vi "USRP Dummy DMA Fixed Fetch (Host).vi"() -> ()   [LabVIEW 2016]
uses:
  <vilib>/userdefined/High Color/nirio_resource_hc.ctl
  <vilib>/FPGAPlugInAG/USRP 294xR; 295xR 200 MSps/niLvFpga_Open_USRP 294xR; 295xR 200 MSps.vi
  <vilib>/rvi/interface/common/dynamic/niFpgaDynamicAddResources.vi
  <vilib>/FPGAPlugInAG/Dynamic/niLvFpga_Download_Dynamic.vi
  <vilib>/FPGAPlugInAG/Dynamic/niLvFpga_Run_Dynamic.vi
  <vilib>/Utility/error.llb/Error Cluster From Error Code.vi
  <vilib>/rvi/errors/niLvFpgaAdjustHostInterfaceError.vi
  <vilib>/rvi/interface/common/niFpgaWaitOnOcc.vi
  <vilib>/FPGAPlugInAG/Dynamic/niLvFpga_Close_Dynamic.vi
  <vilib>/rvi/interface/nirviOpenFPGA/nirviOpenFPGA.xnode
  FPGA Bitfiles/USRP-RIO-Streami_DummyDMA_USRPDummy(FPGA)_kay5ptBR-r4.lvbitx
  <vilib>/rvi/interface/nirviMethod/nirviMethod.xnode
  <vilib>/rvi/interface/nirviReadWriteControl/nirviReadWriteControl.xnode
  <vilib>/rvi/interface/nirviCloseFPGA/nirviCloseFPGA.xnode
  <vilib>/rvi/errors/niLvFpgaMergeErrorWithErrorCode.vi
  <vilib>/rvi/interface/Simulation/niFpgaSimulationCallBeginRW.vi
  <instrlib>/niUsrpRio/Config/v1/Host/niUsrpRio Config v1 Host.lvlib
  NiFpgaLv.dll
  <vilib>/FPGAPlugInAG/Dynamic/niLvFpga_StopFifo_Dynamic.vi
  <vilib>/FPGAPlugInAG/Dynamic/niLvFpga_ConfigureFifo_Dynamic.vi
  <vilib>/FPGAPlugInAG/Dynamic/niLvFpga_StartFifo_Dynamic.vi
  <vilib>/FPGAPlugInAG/Dynamic/niLvFpga_ReadFifo_Dynamic.vi
panel:
  out "Host Transfer Slider":u64(slide) scale=0.0..68719476736.0
  in  "Flush FIFO?":bool
  out "Control Loop":i32
  in  "Host FIFO Fetch":u64=131072
  in  "Reset Host Count?":bool
  in  "Stop Transfer?":bool
  in  "Reset FPGA Count?":bool
  out "FPGA Side FIFO":cluster{u32, u32}(slide)={66, 63} scale=0.0..2047.0
  out "Host Side FIFO":cluster{u32, u32}(slide) scale=0.0..67108863.0
  out "Data Loop":i32
  out "Fetch Loop":i32
  out "Host Transfer Count":u64
  in  "Number of Samples":u64=68719476736
  out "FPGA Transfer Count":u64
  in  "Start Transfer":bool
  in  "stop":bool
  out "Elements Remaining":u32
  out "Data":u64[](array[numeric]) format="%016x"
  out "Timeout Counts":u64
  out "Sticky Timeouts?":bool
  in  "Reset Timeouts?":bool
  out "Actual Depth":u32
  in  "Host Requested Depth":u32=67108864
  out "error out":errorcluster
  in  "error in (no error)":errorcluster
  in  "resource name":T1="PXI2Slot18Port1Dev1"
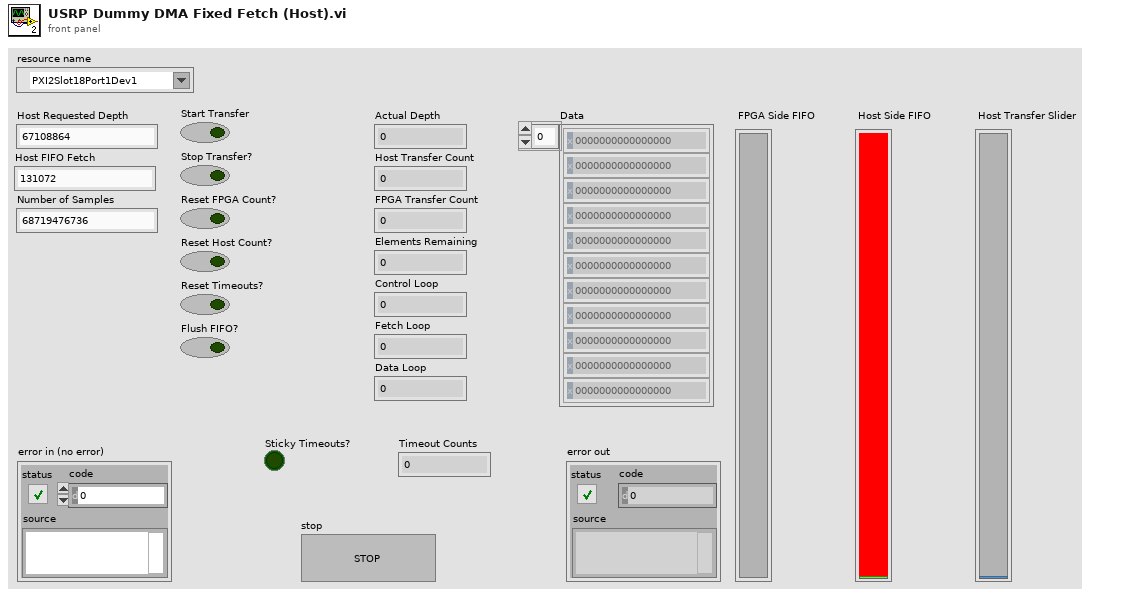
[diagram p1: front panel]
types:
  T1 = typedef "nirio_resource_hc.ctl" = tag
  T2 = typedef "niUsrpRio Config v1 Host.lvlib/niUsrpRio Session.ctl" = cluster{"FPGA Interface":refnum<k20>, "RIO Interface Number":u32, "Data Clock Rate":u32, "FPGA Data Clock Rate":u32, "Global Settings Register Bus":T3, "Radio 0 Settings Register Bus":T3, "Radio 1 Settings Register Bus":T3, "Radio Settings Bus Semaphore":T4, "DB Queues":T5[], "Characterization Data Valid?":bool, "EEPROM Header":T6, "Device Data Header":T7, "EEPROM Characterization Header":T8, "Characterization Data":T9[], "FPGA Current Version":u32, "FPGA Oldest Compatible Version":u32, "Fixed Logic Current Version":u32, "Fixed Logic Oldest Compatible Version":u32, "FPGA Radio Settings Bus Current Version":u32, "FPGA Radio Settings Bus Oldest Compatible Version":u32, "FPGA Board Config Current Version":u32, "FPGA Board Config Oldest Compatible Version":u32, "Daughterboard Clock Rate":u32, "daughterboard configuration session handles":u64[]}
  T3 = typedef "niInstr Register Bus v0 Host.lvlib/Register Bus Session.ctl" = refnum<queue>
  T4 = typedef "Semaphore RefNum" = refnum<k1>
  T5 = typedef "niUsrpRio Config v1 Host.lvlib/DB Queue Reference.ctl" = refnum<queue>
  T6 = typedef "niUsrpRio Config v1 Host.lvlib/EEPROM Header.ctl" = cluster{"Checksum":u32, "Product Code":u16, "Hardware Current Version":u16, "Hardware Oldest Compatible Version":u16, "EEPROM Map Current Version":u16, "EEPROM Map Oldest Compatible Version":u16, "User Password":string, "Pointer to Factory Header":u32, "Pointer to User Header":u32, "Recommended Interval":u16, "Number of Reserved Bytes":i32, "Number of Daughterboards":u8, "Daughterboard IDs":u16[], "Daughterboard Serial Numbers":string[]}
  T7 = typedef "niUsrpRio Config v1 Host.lvlib/EEPROM Device Data Header.ctl" = cluster{"Checksum":u32, "Number of Channels":u8, "Number of Gain Settings":u16[], "Pointer to Characterization Data":u32[], "Number of Reserved Bytes":i32, "Number of Frequencies":u16[]}
  T8 = typedef "niUsrpRio Config v1 Host.lvlib/EEPROM Characterization Header.ctl" = cluster{"Checksum":u32, "Date":timestamp, "Temperature":sgl, "Misc. Info":string, "Pointer to Device Data Header":u32, "Number of Reserved Bytes":i32}
  T9 = typedef "niUsrpRio Config v1 Host.lvlib/Characterization Data.ctl" = cluster{"Gains[dB]":dbl[], "Frequencies [Hz]":dbl[], "IQ Imbalance Table":T10[], "Measured Gains[dB]":dbl[][]}
  T10 = typedef "niUsrpRio Config v1 Host.lvlib/IQ Imbalance.ctl" = cluster{"Gain Imbalance [linear]":dbl, "Phase Imbalance [radians]":dbl, "Offset":cdb}
  T11 = cluster{"Maximum Amount Used":u32, "Current Amount Used":u32}
  T12 = cluster{"Running Max":u32, "Elements Remaining":u32}
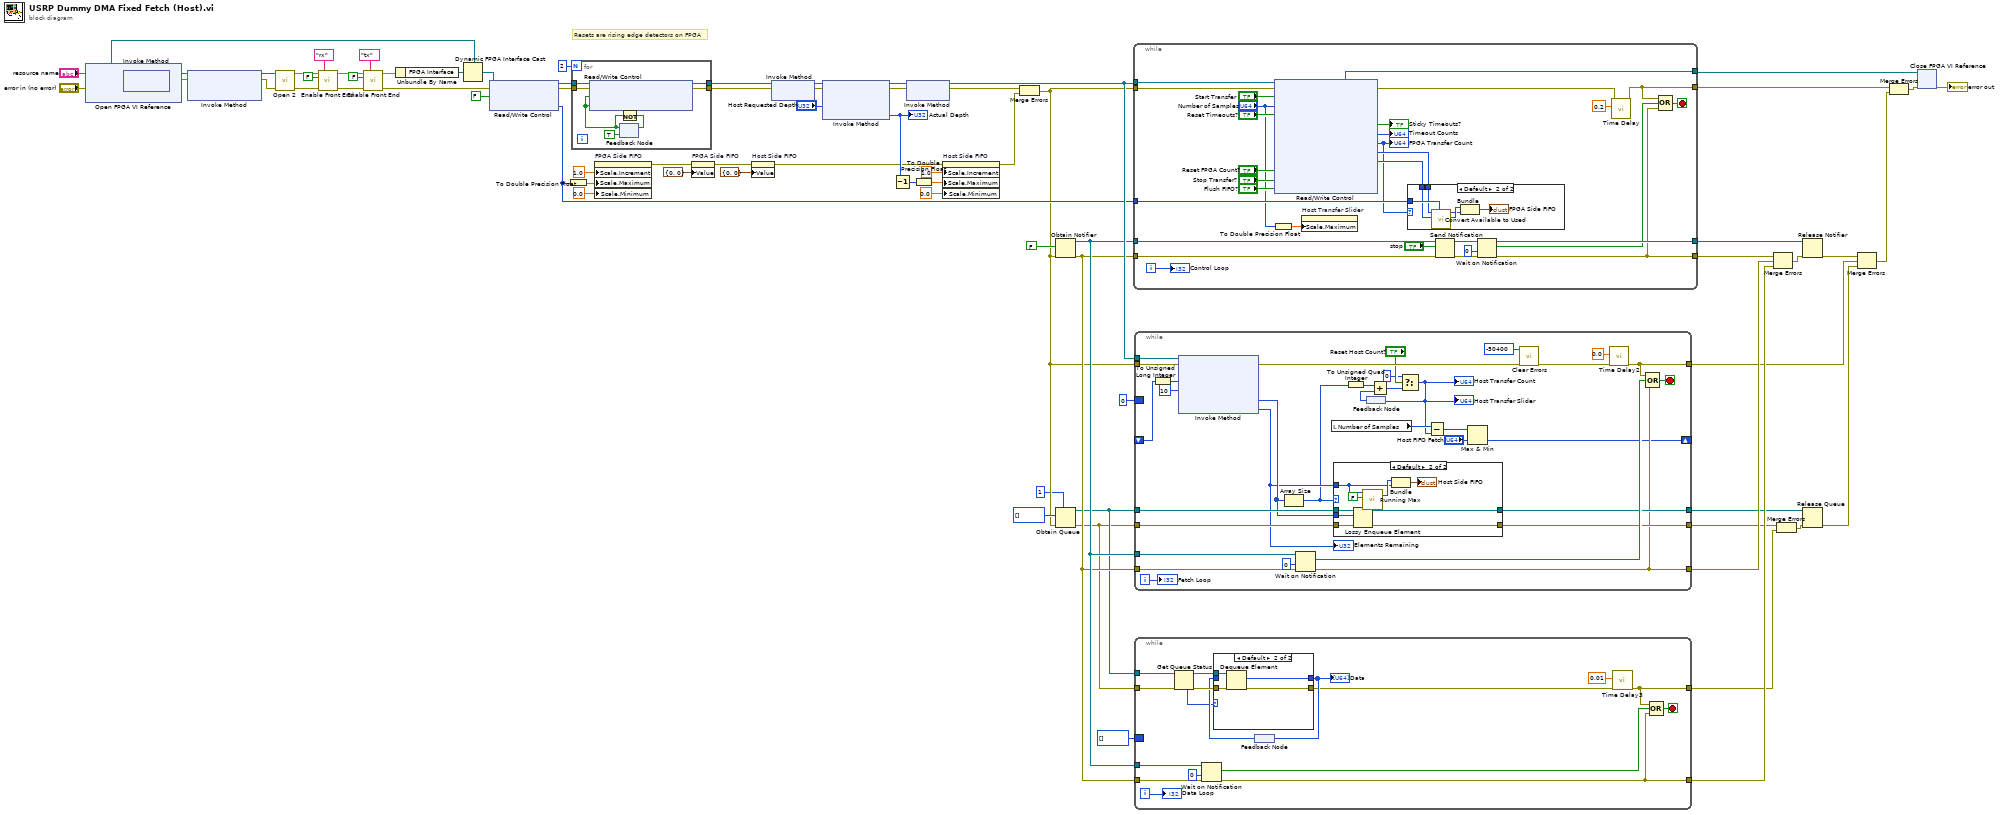
[diagram p0: block diagram]
diagram:
  # "Resets are rising edge detectors on FPGA"
  n1 = xnode "Open FPGA VI Reference"("error in"="error in (no error)", "resource name"="resource name") -> ("FPGA VI Reference Out"=w6:refnum<k20>, "error out"=w5:errorcluster)
  n2 = xnode "Invoke Method"("FPGA VI Reference In"=w6, "error in"=w5) -> ("FPGA VI Reference Out"=w4:refnum<k20>, "error out"=w3:errorcluster)
  n3 = xnode "Invoke Method"("FPGA VI Reference In"=w4, "error in"=w3) -> ("FPGA VI Reference Out"=w2:refnum<k20>, "error out"=w1:errorcluster)  [unwired: 1 in]
  n4 = call <instrlib>:"Open 2.vi"("fpga ref"=w2, "error in"=w1) -> ("niUsrpRio Session (out)"=w64:T2, "error out"=w69:errorcluster)  [unwired: 12 in]
  n5 = call <instrlib>:"Enable Front End.vi"("niUsrpRio Session"=w64, "scope"="rx", "enable"=FALSE, "error in"=w69) -> ("niUsrpRio Session (out)"=w65:T2, "error out"=w68:errorcluster)  [unwired: 10 in]
  n6 = call <instrlib>:"Enable Front End.vi"("niUsrpRio Session"=w65, "scope"="tx", "enable"=FALSE, "error in"=w68) -> ("niUsrpRio Session (out)"=w61:T2, "error out"=w60:errorcluster)  [unwired: 10 in]
  n7 = Unbundle By Name(w61) -> ("FPGA Interface"=w59:refnum<k20>)
  n8 = Dynamic FPGA Interface Cast(Session In=w6, Type=w59) -> (Session Out=w58:refnum<k20>)
  n9 = xnode "Read/Write Control"("FPGA VI Reference In"=w58, "error in"=w60, "Start Transfer?"=FALSE ("send data?")) -> ("FPGA VI Reference Out"=w35:refnum<k20>, "error out"=w34:errorcluster, "FPGA FIFO Depth"=w20:u32)
  n10 = To Double Precision Float(number=w20) -> (double precision float=w22:dbl)
  n11 = for {
    N: 2 -> [_]
    tunnel: w35 -> [w82]
    tunnel: w34 -> [w81]
    tunnel: [w80] -> w33
    tunnel: [w79] -> w32
    n12 = feedback #1(TRUE) -> (w77:bool)
    n13 = xnode "Read/Write Control"("FPGA VI Reference In"=w82, "error in"=w81, "Reset Total Timeouts?"=w77, "Reset FPGA Transfer Count?"=w77) -> ("FPGA VI Reference Out"=w80:refnum<k20>, "error out"=w79:errorcluster)
    n14 = Not(x=w77) -> (.not. x?=w76:bool)
    n15 = feedback-in #1(w76) -> ()
  }
  n16 = property on="FPGA Side FIFO" class="Slide (strict)"("Scale.Increment"=1.0 ("Scale.Range:Increment"), "Scale.Maximum"=w22, "Scale.Minimum"=0.0 ("Scale.Range:Minimum")) -> (error out=w15:errorcluster)  [unwired: 2 in, 1 out]
  n17 = property on="FPGA Side FIFO" class="Slide (strict)"(error in=w15, "Value"=cluster{u32, u32} {0, 0} ("FPGA Side FIFO")) -> (error out=w18:errorcluster)  [unwired: 1 in, 1 out]
  n18 = property on="Host Side FIFO" class="Slide (strict)"(error in=w18, "Value"=cluster{u32, u32} {0, 0} ("FPGA Side FIFO")) -> (error out=w14:errorcluster)  [unwired: 1 in, 1 out]
  n19 = xnode "Invoke Method"("FPGA VI Reference In"=w33, "error in"=w32) -> ("FPGA VI Reference Out"=w75:refnum<k20>, "error out"=w74:errorcluster)
  n20 = xnode "Invoke Method"("FPGA VI Reference In"=w75, "error in"=w74, "Requested Depth"="Host Requested Depth") -> ("FPGA VI Reference Out"=w71:refnum<k20>, "error out"=w72:errorcluster, "Actual Depth"=w19:u32)
  "Actual Depth" <- w19
  n21 = Decrement(x=w19) -> (x-1=w25:u32)
  n22 = xnode "Invoke Method"("FPGA VI Reference In"=w71, "error in"=w72) -> ("FPGA VI Reference Out"=w55:refnum<k20>, "error out"=w21:errorcluster)
  n23 = To Double Precision Float(number=w25) -> (double precision float=w7:dbl)
  n24 = property on="Host Side FIFO" class="Slide (strict)"(error in=w14, "Scale.Increment"=1.0 ("Data Entry Limits:Increment"), "Scale.Maximum"=w7, "Scale.Minimum"=0.0 ("Data Entry Limits:Minimum")) -> (error out=w12:errorcluster)  [unwired: 1 in, 1 out]
  n25 = Merge Errors(w21, w12) -> (w13:errorcluster)
  n26 = Obtain Notifier(notification data type=FALSE, error in (no error)=w13) -> (notifier out=w47:refnum<notifier>, error out=w46:errorcluster)  [unwired: 2 in, 1 out]
  n27 = Obtain Queue(max queue size (-1, unlimited)=1, element data type=u64[] [] ("Data"), error in (no error)=w13) -> (queue out=w39:refnum<queue>, error out=w38:errorcluster)  [unwired: 2 in, 1 out]
  n28 = while {
    tunnel: w55 -> [w112]
    tunnel: w13 -> [w111]
    tunnel: w47 -> [w108]
    tunnel: w46 -> [w107]
    tunnel: [w102] -> w52
    tunnel: [w94] -> w51
    tunnel: [w96] -> w30
    tunnel: [w95] -> w29
    tunnel: w20 -> [w93]
    i -> [w86]
    stop <- w101 stop-if-true
    n29 = xnode "Read/Write Control"("FPGA VI Reference In"=w112, "error in"=w111, "Start Transfer?"="Start Transfer", "Number of Samples"="Number of Samples", "Reset Total Timeouts?"="Reset Timeouts?", "Reset FPGA Transfer Count?"="Reset FPGA Count?", "Stop Transfer?"="Stop Transfer?", "Flush FIFO?"="Flush FIFO?") -> ("FPGA VI Reference Out"=w95:refnum<k20>, "error out"=w110:errorcluster, "Sticky Timeout?"=→"Sticky Timeouts?":bool, "Timeout Count"=→"Timeout Counts":u64, "FPGA Transfer Count"=w87:u64, "Space Available"=w92:u32, "Min Space Available"=w90:u32)
    "FPGA Transfer Count" <- w87
    n30 = To Double Precision Float(number="Number of Samples") -> (double precision float=w83:dbl)
    n31 = property on="Host Transfer Slider" class="Slide (strict)"("Scale.Maximum"=w83) -> ()  [unwired: 2 in, 2 out]
    n32 = case shown="Default" w87 {
      tunnel: w93 -> [_ w118]
      tunnel: w92 -> [_ w117]
      tunnel: w90 -> [_ w116]
      frame 0 {
      }
      frame Default {
        n33 = call "Convert Available to Used.vi"("Size"=w118, "Minimum Amount Available"=w116, "Current Amount Available"=w117) -> ("Maximum Amount Used"=w115:u32, "Current Amount Used"=w114:u32)  [unwired: 5 in]
        n34 = Bundle("Maximum Amount Used"=w115, "Current Amount Used"=w114) -> (→"FPGA Side FIFO":T11)  [unwired: 1 in]
      }
    }
    n35 = Send Notification(notification="stop", notifier=w108, error in (no error)=w107) -> (notifier out=w104:refnum<notifier>, error out=w103:errorcluster)
    n36 = Wait on Notification(notifier=w104, timeout in ms (-1)=0, error in (no error)=w103) -> (notifier out=w102:refnum<notifier>, notification=w100:bool, error out=w94:errorcluster)  [unwired: 1 in, 1 out]
    n37 = call "Time Delay"("error in (no error)"=w110, "Delay Time (s)"=0.2) -> ("error out"=w96:errorcluster)  [unwired: 9 in]
    n38 = Compound Arithmetic op=OR(w96, w100, w94) -> (w101:bool)
    "Control Loop" <- w86
  }
  n39 = while {
    tunnel: [w147] -> w31
    tunnel: w55 -> [w150]
    tunnel: w13 -> [w149]
    border: u64 0 -> [_]
    tunnel: w47 -> [w143]
    tunnel: w46 -> [w142]
    tunnel: [w133] -> w49
    tunnel: [w138] -> w43
    tunnel: w39 -> [w139]
    tunnel: w38 -> [w137]
    tunnel: [w136] -> w42
    shift-right: [w123] -> _
    shift-left: _ -> [w124]
    i -> [w140]
    stop <- w145 stop-if-true
    n40 = To Unsigned Long Integer(number=w124) -> (unsigned 32bit integer=w122:u32)
    n41 = xnode "Invoke Method"("FPGA VI Reference In"=w150, "error in"=w149, "Number of Elements"=w122, "Timeout (ms)"=10) -> ("error out"=w135:errorcluster, "Data"=w134:u64[], "Elements Remaining"=w129:u32)  [unwired: 1 out]
    "Elements Remaining" <- w129
    n42 = Array Size(array=w134) -> (size(s)=w128:i32)
    n43 = Wait on Notification(notifier=w143, timeout in ms (-1)=0, error in (no error)=w142) -> (notification=w141:bool, error out=w133:errorcluster)  [unwired: 1 in, 2 out]
    n44 = local read "Number of Samples"() -> (w127:u64)
    n45 = case shown="Default" w128 {
      tunnel: w139 -> [w154 w163]
      tunnel: [w154 w162] -> w138
      tunnel: w137 -> [w153 w161]
      tunnel: [w153 w160] -> w136
      tunnel: w134 -> [_ w159]
      tunnel: w129 -> [_ w155]
      frame 0 {
      }
      frame Default {
        n46 = Lossy Enqueue Element(queue=w163, element=w159, error in (no error)=w161) -> (queue out=w162:refnum<queue>, error out=w160:errorcluster)  [unwired: 2 out]
        n47 = call "Running Max.vi"("Reset"=FALSE, "Next Value"=w155) -> ("Running Max"=w156:u32)  [unwired: 5 in]
        n48 = Bundle("Running Max"=w156, "Elements Remaining"=w155) -> (→"Host Side FIFO":T12)  [unwired: 1 in]
      }
    }
    n49 = To Unsigned Quad Integer(1:w128) -> (0:w152:u64)
    n50 = feedback #2() -> (w151:u64)
    n51 = Add(x=w152, y=w151) -> (x+y=w131:u64)
    n52 = Select(t=u64 0, s="Reset Host Count?", f=w131) -> (s? t:f=w126:u64)
    "Host Transfer Count" <- w126
    "Host Transfer Slider" <- w126
    n53 = feedback-in #2(w126) -> ()
    n54 = Subtract(x=w127, y=w126) -> (x-y=w125:u64)
    n55 = Max & Min(x=w125, y="Host FIFO Fetch") -> (min(x,y)=w123:u64)  [unwired: 1 out]
    n56 = call <vilib>:"Clear Errors.vi"("error in (no error)"=w135, "specific error code to clear (0: all)"=-50400) -> ("error out"=w121:errorcluster)  [unwired: 4 in, 1 out]
    n57 = call "Time Delay2"("error in (no error)"=w121, "Delay Time (s)"=0.0) -> ("error out"=w147:errorcluster)  [unwired: 9 in]
    n58 = Compound Arithmetic op=OR(w147, w141, w133) -> (w145:bool)
    "Fetch Loop" <- w140
  }
  n59 = while {
    tunnel: w47 -> [w178]
    tunnel: w46 -> [w177]
    tunnel: [w164] -> w45
    tunnel: w39 -> [w175]
    tunnel: w38 -> [w174]
    tunnel: [w166] -> w37
    border: u64[] [] -> [_]
    i -> [w180]
    stop <- w168 stop-if-true
    n60 = Get Queue Status(queue=w175, error in (no error)=w174) -> (queue out=w172:refnum<queue>, error out=w173:errorcluster, # elements in queue=w169:i32)  [unwired: 1 in, 5 out]
    n61 = Wait on Notification(notifier=w178, timeout in ms (-1)=0, error in (no error)=w177) -> (notification=w176:bool, error out=w164:errorcluster)  [unwired: 1 in, 2 out]
    n62 = feedback #3() -> (w171:u64[])
    n63 = case shown="Default" w169 {
      tunnel: [w182 w186] -> w167
      tunnel: [w181 w183] -> w170
      tunnel: w173 -> [w182 w185]
      tunnel: w172 -> [_ w184]
      tunnel: w171 -> [w181 _]
      frame 0 {
      }
      frame Default {
        n64 = Dequeue Element(queue=w184, error in (no error)=w185) -> (element=w183:u64[], error out=w186:errorcluster)  [unwired: 1 in, 2 out]
      }
    }
    "Data" <- w170
    n65 = feedback-in #3(w170) -> ()
    n66 = call "Time Delay3"("error in (no error)"=w167, "Delay Time (s)"=0.01) -> ("error out"=w166:errorcluster)  [unwired: 9 in]
    n67 = Compound Arithmetic op=OR(w166, w176, w164) -> (w168:bool)
    "Data Loop" <- w180
  }
  n68 = Merge Errors(w51, w49, w45) -> (w50:errorcluster)
  n69 = Merge Errors(w42, w37) -> (w41:errorcluster)
  n70 = Release Notifier(notifier=w52, error in (no error)=w50) -> (error out=w48:errorcluster)  [unwired: 1 in, 2 out]
  n71 = Release Queue(queue=w43, error in (no error)=w41) -> (error out=w40:errorcluster)  [unwired: 1 in, 2 out]
  n72 = Merge Errors(w48, w31, w40) -> (w8:errorcluster)
  n73 = Merge Errors(w30, w8) -> (w9:errorcluster)
  n74 = xnode "Close FPGA VI Reference"("FPGA VI Reference In"=w29, "error in"=w9) -> ("error out"=→"error out":errorcluster)
